vi "GV stage z position.vi"() -> ()   [LabVIEW 2017]
panel:
  out "StageZposition":bool
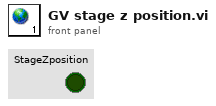
[diagram p1: front panel]
diagram:
